vi "writeMultiBuffer.vi"(0 "Corresponding channels":i32[](array[numeric]), 1 "storage paths":string[](array[string])=["Storage path", "", "", "", "", "", "", "", "", "", "", "", "", "", ""], 2 "comment":string, 3 "binary":bool, 4 "fwd&bwd?":bool, 5 "error in":T1) -> (19 "error out":T1)   [LabVIEW 2016]
doc: "Writes the data points of the channels into a asc-file.The inputs are:\n- Corresponding channels: This array contains channel numbers. The data, that can be retrieved from these channels, will be saved into the output-file.\n- fileName: This input is is of type string. The output-file will be named like the string entered here. Furthermore a path can be entered and the output file will be saved to the desired path.\n- Comment: You can add a comment to the output file. It can be found in the header of the file.\n- Binary: If this input is \"false\" the output file will be of type .asc. If it is \"true\" the output file will be of type .bcrf."
uses:
  Controls/Error_Out.ctl
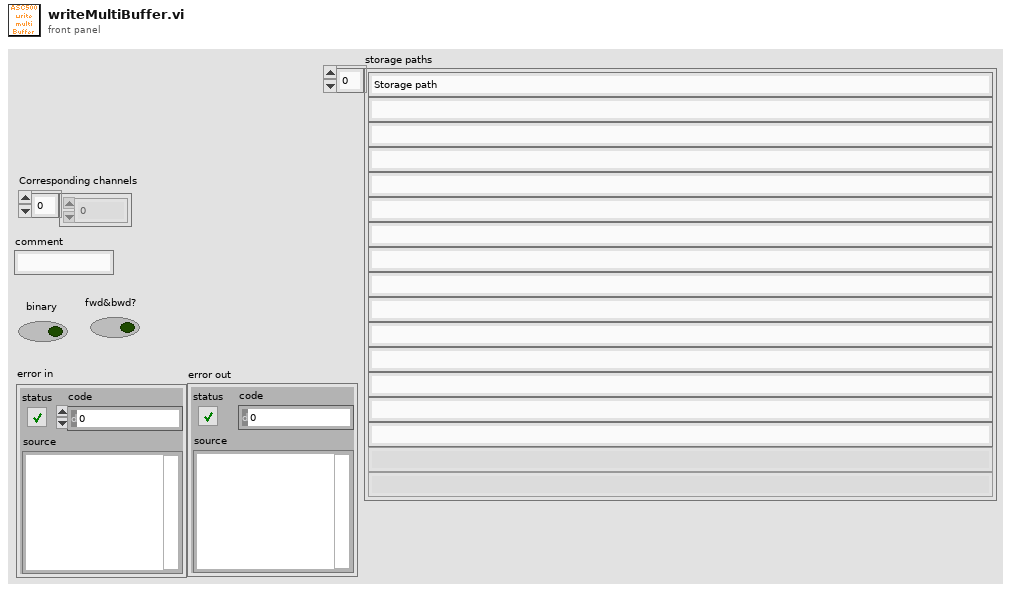
[diagram p1: front panel]
types:
  T1 = typedef "Error_Out.ctl" = errorcluster
  T2 = typedef "Metadata-Cluster.ctl" = cluster{"DYB_Order":i32, "Spalte":i32, "Zeile":i32, "Abstand Datenpunkte":dbl, "Abstand Scanzeilen":dbl, "x-Koordinate 1. Punkt":dbl, "y-Koordinate 2. Punkt":dbl, "Neigungswinkel Scanfeld":dbl, "Einheit Variablen":i32, "stepVal":dbl, "stepValNum":dbl, "offsetVal":dbl, "unitVal":i32}
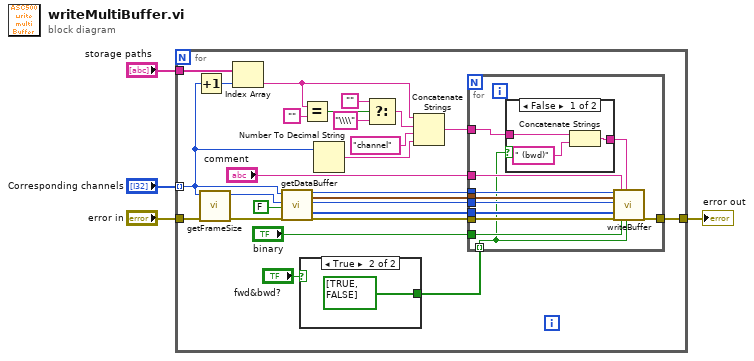
[diagram p0: block diagram]
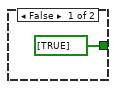
[diagram p2: hidden frame]
diagram:
  n1 = for {
    tunnel: [w29] -> w4
    tunnel: "Corresponding channels" -> [w13] mode=indexing
    tunnel: "error in" -> [w27]
    tunnel: "storage paths" -> [w16]
    n2 = Increment(x=w13) -> (x+1=w12:i32)
    n3 = call "getFrameSize.vi"("error in"=w27, "channel"=w13) -> ("error out"=w26:T1, "FrameSize"=w25:i32)  [unwired: 8 in]
    n4 = Index Array(array=w16, index=w12) -> (element=w5:string)
    n5 = call "getDataBuffer.vi"("channel"=w13, "dataSize_in"=w25, "FullOnly"=FALSE, "error in"=w26) -> ("dataSize"=w23:i32, "meta"=w22:T2, "indexinit"=w21:i32, "data"=w20:i32[], "error out"=w30:T1)  [unwired: 10 in, 1 out]
    n6 = case shown="True" "fwd&bwd?" {
      tunnel: [bool[] [TRUE] bool[] [TRUE, FALSE]] -> w19
      frame False {
      }
      frame True {
      }
    }
    n7 = Equal?(x=w5, y="") -> (x = y?=w9:bool)
    n8 = Number To Decimal String(number=w13) -> (decimal integer string=w11:string)  [unwired: 1 in]
    n9 = Select(t="", s=w9, f="\\\\" ("string")) -> (s? t:f=w6:string)
    n10 = Concatenate Strings(w5, w6, "channel" ("string"), w11) -> (w15:string)
    n11 = for {
      tunnel: w30 -> [w43]
      tunnel: [w42] -> w29
      tunnel: "binary" -> [w41]
      tunnel: w23 -> [w40]
      tunnel: w22 -> [w39]
      tunnel: w21 -> [w38]
      tunnel: w20 -> [w37]
      tunnel: w19 -> [w33] mode=indexing
      tunnel: "comment" -> [w36]
      tunnel: w15 -> [w35]
      n12 = case shown="False" w33 {
        tunnel: w35 -> [w46 w47]
        tunnel: [w45 w47] -> w34
        frame False {
          n13 = Concatenate Strings(w46, " (bwd)") -> (w45:string)
        }
        frame True {
        }
      }
      n14 = call "writeBuffer.vi"("dataSize"=w40, "meta"=w39, "index"=w38, "data"=w37, "error in"=w43, "comment"=w36, "binary"=w41, "fileName"=w34, "forward"=w33) -> ("error out"=w42:T1)  [unwired: 10 in]
    }
  }
  "error out" <- w4
